vi "dfd_Sort Zeros based on Modulus.vi"(11 "zeros":cdb[](array[numeric])) -> (1 ">1":cdb[](array[numeric]), 2 "=1":cdb[](array[numeric]), 3 "<1":cdb[](array[numeric]))   [LabVIEW 2017, in "NI_DigFilter_Design.lvlib"]
doc: "Classifies the input zeros by comparing its modulus with 1."
uses:
  <vilib>/addons/Digital Filter Design/NI_DigFilter_Design.lvlib
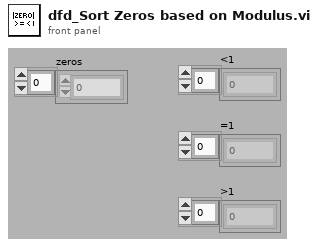
[diagram p1: front panel]
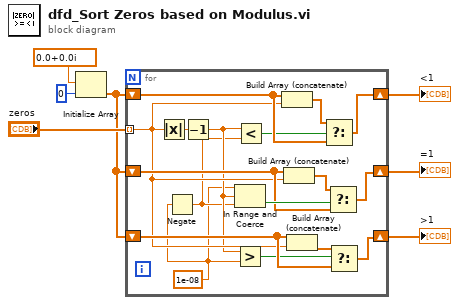
[diagram p0: block diagram]
diagram:
  n1 = Initialize Array(cdb 0.0+0.0i, 0) -> (w1:cdb[])
  n2 = for {
    tunnel: "zeros" -> [w11] mode=indexing
    shift-right: [w23] -> w4
    shift-left: w1 -> [w24]
    shift-right: [w22] -> w5
    shift-left: w1 -> [w21]
    shift-right: [w12] -> w7
    shift-left: w1 -> [w13]
    w8 = 1e-08
    n3 = Absolute Value(x=w11) -> (abs(x)=w16:dbl)
    n4 = Negate(x=w8) -> (-x=w9:dbl)
    n5 = Decrement(x=w16) -> (x-1=w10:dbl)
    n6 = In Range and Coerce(upper limit=w8, x=w10, lower limit=w9) -> (In Range?=w15:bool)  [unwired: 1 out]
    n7 = Greater?(x=w10, y=w8) -> (0:w18:bool)
    n8 = Less?(x=w10, y=w9) -> (x < y?=w20:bool)
    n9 = Build Array (concatenate)(w24, w11) -> (w19:cdb[])
    n10 = Build Array (concatenate)(w13, w11) -> (w14:cdb[])
    n11 = Build Array (concatenate)(w21, w11) -> (w17:cdb[])
    n12 = Select(t=w19, s=w20, f=w24) -> (s? t:f=w23:cdb[])
    n13 = Select(t=w14, s=w15, f=w13) -> (s? t:f=w12:cdb[])
    n14 = Select(t=w17, s=w18, f=w21) -> (s? t:f=w22:cdb[])
  }
  "=1" <- w7
  ">1" <- w5
  "<1" <- w4
